vi "resultShow.vi"() -> ()   [LabVIEW 2013]
panel:
  in  "runMode 2":bool
  out "countRight":refnum<vi>
  out "countLeft":refnum<vi>
  in  "TblRefFormMainPar2":refnum<vi>
  in  "TblRefFormMainPar1":refnum<vi>
  out "Status":T1
  out "LED":refnum<vi>[](array[refnum])
  out "Ring":refnum<vi>
  out "Tab":refnum<vi>
  in  "runMode":refnum<vi>
  in  "XYGraphTXCGQ":refnum<vi>
  in  "XYGraphTXDL":refnum<vi>
  in  "XYGraphNKZ":refnum<vi>
  in  "XYGraphKZ":refnum<vi>
  in  "XYGraphTXSS":refnum<vi>
  in  "TblRefFormAlarmUnchecked":refnum<vi>
  in  "WFGraph引用句柄Order":refnum<vi>
  in  "WFGraph引用句柄FFT":refnum<vi>
  in  "TblRefFormMainShow":refnum<vi>
  in  "XYGraphGN":refnum<vi>
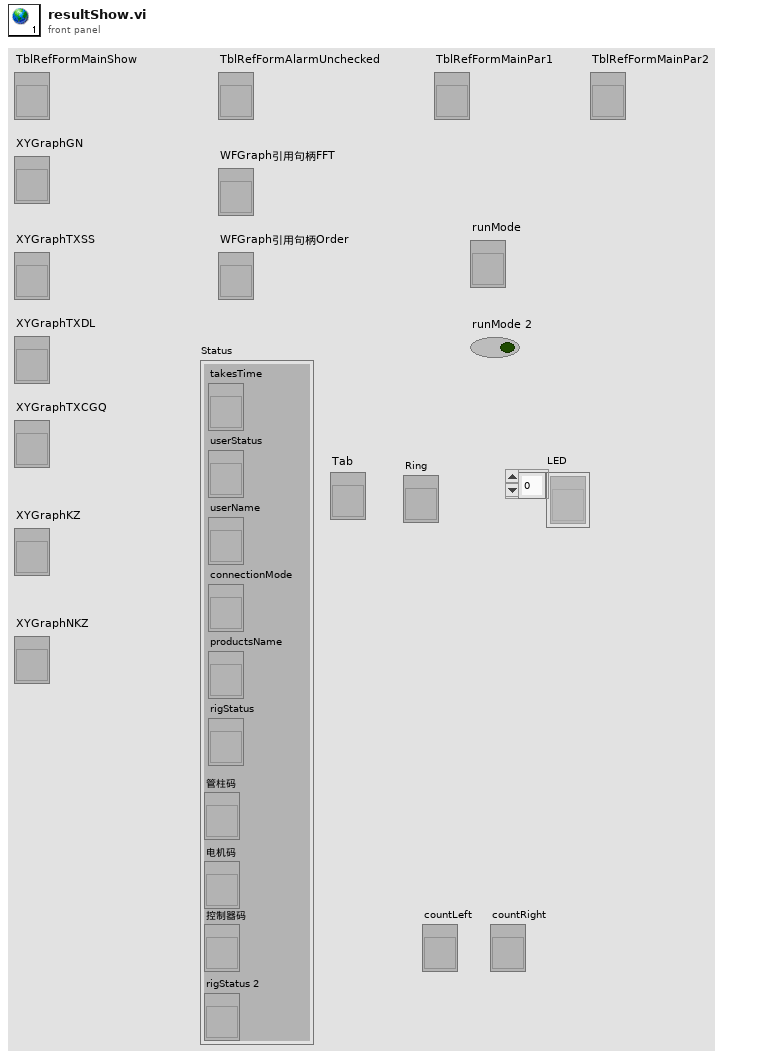
[diagram p1: front panel]
types:
  T1 = cluster{"takesTime":refnum<vi>, "userStatus":refnum<vi>, "userName":refnum<vi>, "connectionMode":refnum<vi>, "productsName":refnum<vi>, "rigStatus":refnum<vi>, "管柱码":refnum<vi>, "电机码":refnum<vi>, "控制器码":refnum<vi>, "rigStatus 2":refnum<vi>}
diagram:
